vi "ProfiledPIDController_GetSetpoint.vi"(11 "in PROFILED_PID_CONTROLLER":T2={"Controller"={"Kp"=0.0, "Ki"=0.0, "Kd"=0.0, "Period"=0.0, "Max_Integral"=1.0, "Min_Integral"=-1.0, "Max_Input"=0.0, "Min_Input"=0.0, "Continuous"=FALSE, "PositionError"=0.0, "VelocityError"=0.0, "PrevError"=0.0, "TotalError"=0.0, "PositionTolerance"=0.05, "VelocityTolerance"=9.99e+35, "SetPoint"=0.0, "Kf"=0.0, "Prev_Deriv"=0.0, "Prev_Deriv 2"=0.0, "DerivativeFilter"=FALSE, "Min_Output"=-9.99e+35, "Max_Output"=9.9e+35, "Prev_F_P"=0.0, "Prev_F_P_2"=0.0, "AntiWindupActive"=FALSE}, "Goal"={"Position"=0.0, "Velocity"=0.0}, "Setpoint"={"Position"=0.0, "Velocity"=0.0}, "Constraint"={"MaxVelocity"=0.0, "MaxAcceleration"=0.0}} {"Constraint"."MaxAcceleration" format="%16_6e"; "Constraint"."MaxVelocity" format="%16_6e"; "Setpoint"."Velocity" format="%16_6e"; "Setpoint"."Position" format="%16_6e"; "Goal"."Velocity" format="%16_6e"; "Goal"."Position" format="%16_6e"; "Controller"."Prev_F_P_2" format="%16_6e"; "Controller"."Prev_F_P" format="%16_6e"; "Controller"."Max_Output" format="%16_6e"; "Controller"."Min_Output" format="%16_6e"; "Controller"."Prev_Deriv 2" format="%16_6e"; "Controller"."Prev_Deriv" format="%16_6e"; "Controller"."Kf" format="%16_6e"; "Controller"."SetPoint" format="%16_6e"; "Controller"."VelocityTolerance" format="%16_6e"; "Controller"."PositionTolerance" format="%16_6e"; "Controller"."TotalError" format="%16_6e"; "Controller"."PrevError" format="%16_6e"; "Controller"."VelocityError" format="%16_6e"; "Controller"."PositionError" format="%16_6e"; "Controller"."Min_Input" format="%16_6e"; "Controller"."Max_Input" format="%16_6e"; "Controller"."Min_Integral" format="%16_6e"; "Controller"."Max_Integral" format="%16_6e"; "Controller"."Period" format="%16_6e"; "Controller"."Kd" format="%16_6e"; "Controller"."Ki" format="%16_6e"; "Controller"."Kp" format="%16_6e"}) -> (3 "Setpoint":T1 {"Velocity" format="%16_6e"; "Position" format="%16_6e"})   [LabVIEW 2019, in "Trajectory_Library.lvlib"]
doc: "Returns the current setpoint of the ProfiledPIDController.\n\nInputs:\n - Profiled_PID_Controller -- Profiled_PID_Controller data cluster\n\nOutputs:\n - Setpoint -- The current setpoint, returned as a Trapezoid Profile State data cluster"
uses:
  Trajectory_Library.lvlib
  PROFILED_PID_CONTROLLER.ctl
  PID_CONTROLLER.ctl
  TRAPEZOID_PROFILE_STATE.ctl
  TRAPEZOID_PROFILE_CONSTRAINT.ctl
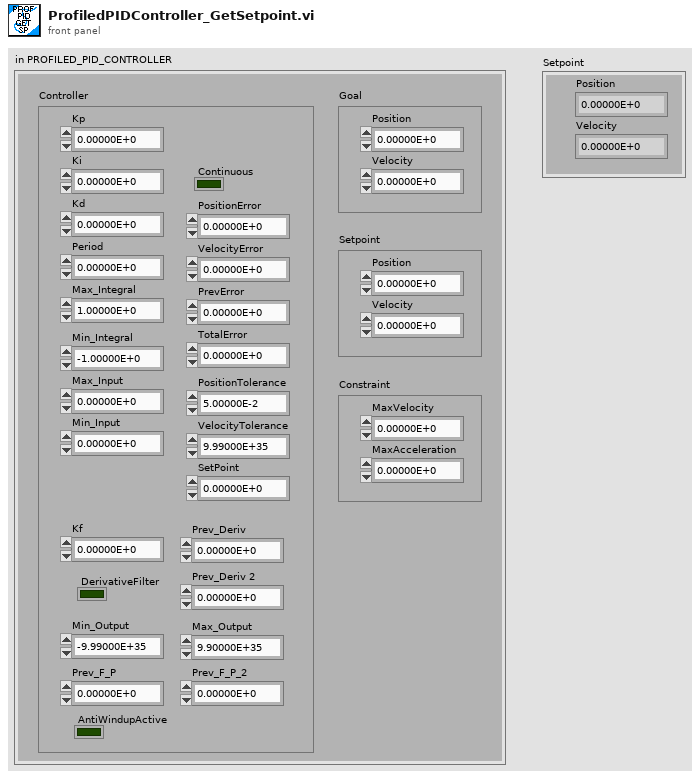
[diagram p1: front panel]
types:
  T1 = typedef "Trajectory_Library.lvlib/TRAPEZOID_PROFILE_STATE.ctl" = cluster{"Position":dbl, "Velocity":dbl}
  T2 = typedef "Trajectory_Library.lvlib/PROFILED_PID_CONTROLLER.ctl" = cluster{"Controller":T3, "Goal":T1, "Setpoint":T1, "Constraint":T4}
  T3 = typedef "Trajectory_Library.lvlib/PID_CONTROLLER.ctl" = cluster{"Kp":dbl, "Ki":dbl, "Kd":dbl, "Period":dbl, "Max_Integral":dbl, "Min_Integral":dbl, "Max_Input":dbl, "Min_Input":dbl, "Continuous":bool, "PositionError":dbl, "VelocityError":dbl, "PrevError":dbl, "TotalError":dbl, "PositionTolerance":dbl, "VelocityTolerance":dbl, "SetPoint":dbl, "Kf":dbl, "Prev_Deriv":dbl, "Prev_Deriv 2":dbl, "DerivativeFilter":bool, "Min_Output":dbl, "Max_Output":dbl, "Prev_F_P":dbl, "Prev_F_P_2":dbl, "AntiWindupActive":bool}
  T4 = typedef "Trajectory_Library.lvlib/TRAPEZOID_PROFILE_CONSTRAINT.ctl" = cluster{"MaxVelocity":dbl, "MaxAcceleration":dbl}
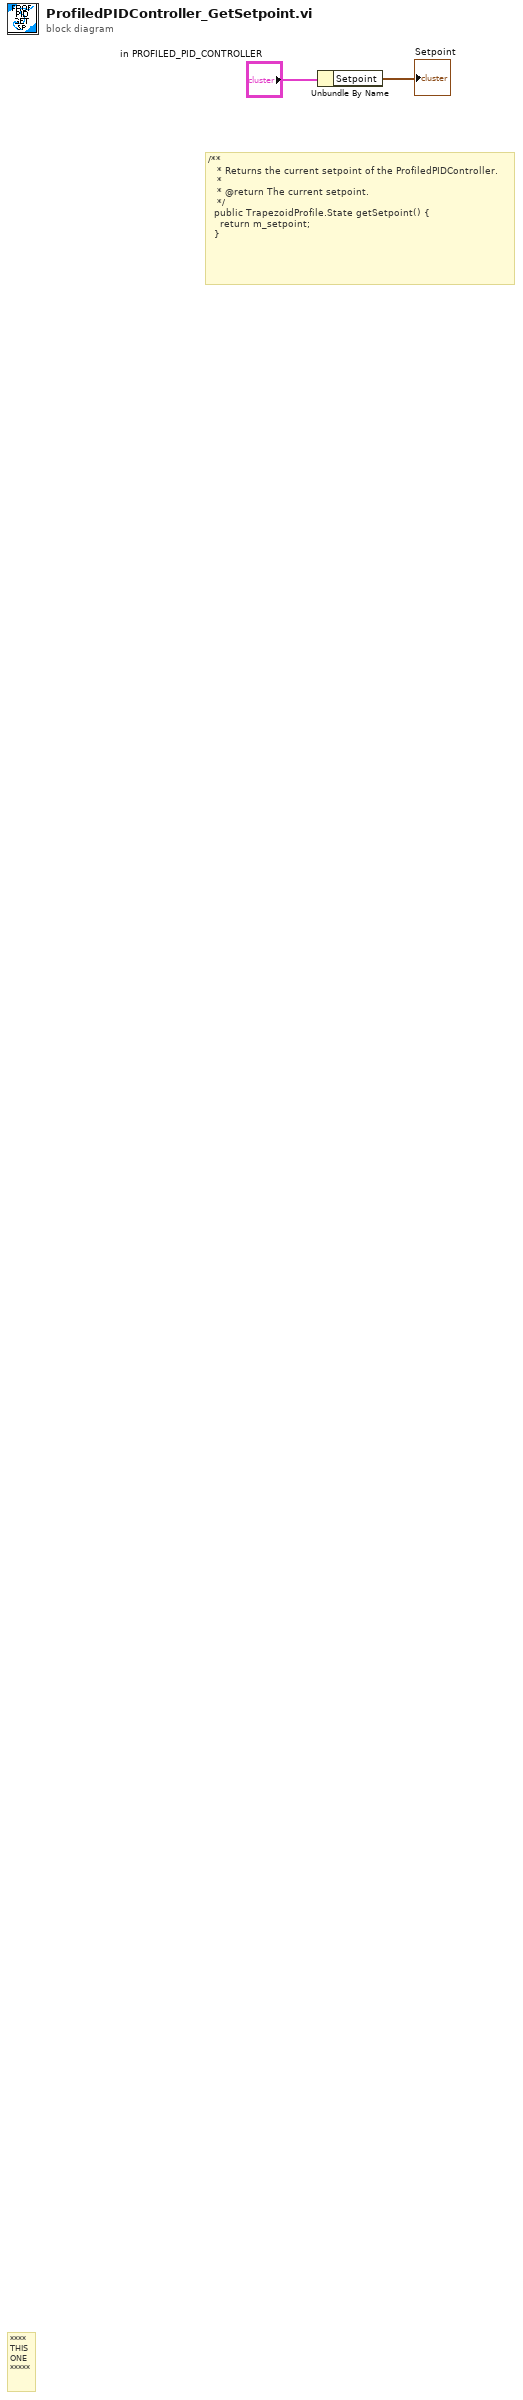
[diagram p0: block diagram]
diagram:
  # "/**\n   * Returns the current setpoint of the ProfiledPIDController.\n   *\n   * @return The current setpoint.\n   */\n  public TrapezoidProfile.State getSetpoint() {\n    return m_setpoint;\n  }"
  # "****\nTHIS\nONE\n*****"
  n1 = Unbundle By Name("in PROFILED_PID_CONTROLLER") -> ("Setpoint"=→"Setpoint":T1)
